vi "Adjust and Check Bounds.vi"(10 "GUI Properties":T1, 11 "Saved Bounds":T2) -> (2 "Center":bool, 3 "Bounds":T2)   [LabVIEW 2020, in "VolatusGUI.lvlib" / "GUI Helper.lvclass"]
uses:
  GUI Helper.lvclass
  <vilib>/Utility/miscctls.llb/LVRectTypeDef.ctl
  GUI Properties.ctl
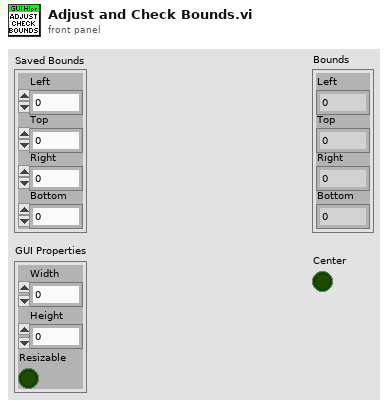
[diagram p1: front panel]
types:
  T1 = typedef "VolatusGUI.lvlib/GUI Helper.lvclass/GUI Properties.ctl" = cluster{"Width":u16, "Height":u16, "Resizable":bool}
  T2 = typedef "LVRectTypeDef.ctl" = cluster{"Left":i16, "Top":i16, "Right":i16, "Bottom":i16}
  T3 = typedef "LVAllMonitorsDisplayTypeDef.ctl" = cluster{"Bounds":cluster{"Left":i16, "Top":i16, "Right":i16, "Bottom":i16}, "Depth":i16}[]
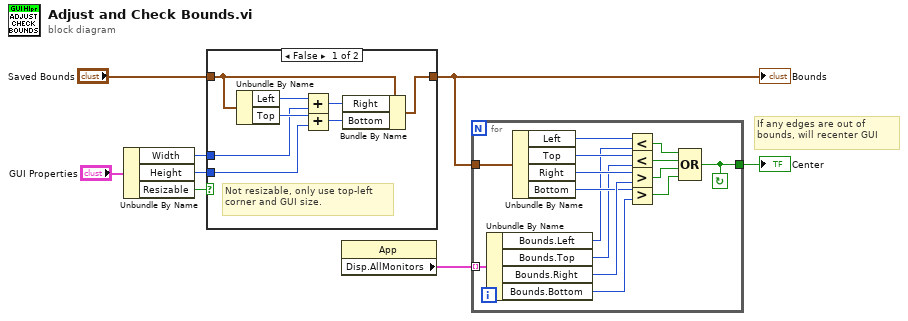
[diagram p0: block diagram]
diagram:
  # "If any edges are out of bounds, will recenter GUI"
  n1 = Unbundle By Name("GUI Properties") -> ("Width"=w6:u16, "Height"=w5:u16, "Resizable"=w7:bool)
  n2 = case shown="False" w7 {
    tunnel: w6 -> [w14 _]
    tunnel: w5 -> [w13 _]
    tunnel: "Saved Bounds" -> [w12 w17]
    tunnel: [w9 w17] -> w2
    frame False {
      # "Not resizable, only use top-left corner and GUI size."
      n3 = Unbundle By Name(w12) -> ("Left"=w16:i16, "Top"=w15:i16)
      n4 = Add(x=w16, y=w14) -> (x+y=w11:u16)
      n5 = Add(x=w15, y=w13) -> (x+y=w10:u16)
      n6 = Bundle By Name(cluster=w12, "Right"=w11, "Bottom"=w10) -> (w9:T2)
    }
    frame True {
      # "Resizable, use bounds as-is"
    }
  }
  "Bounds" <- w2
  n7 = property class="App"() -> ("Disp.AllMonitors"=w3:T3)  [unwired: 2 in, 2 out]
  n8 = for {
    tunnel: w2 -> [w31]
    tunnel: w3 -> [w32] mode=indexing
    tunnel: [w18] -> w1
    stop <- w18 continue-if-true
    n9 = Unbundle By Name(w32) -> ("Bounds.Left"=w23:i16, "Bounds.Top"=w24:i16, "Bounds.Right"=w29:i16, "Bounds.Bottom"=w27:i16)
    n10 = Unbundle By Name(w31) -> ("Left"=w25:i16, "Top"=w26:i16, "Right"=w30:i16, "Bottom"=w28:i16)
    n11 = Less?(x=w25, y=w23) -> (x < y?=w19:bool)
    n12 = Less?(x=w26, y=w24) -> (x < y?=w22:bool)
    n13 = Greater?(x=w30, y=w29) -> (0:w21:bool)
    n14 = Greater?(x=w28, y=w27) -> (0:w20:bool)
    n15 = Compound Arithmetic op=OR(w19, w22, w21, w20) -> (w18:bool)
  }
  "Center" <- w1
